vi "Queues Init.vi"(8 "error in (no error)":errorcluster, 11 "Guardian in":refnum<class "Guardian.lvclass">) -> (0 "error out":errorcluster, 3 "Guardian out":refnum<class "Guardian.lvclass">)   [LabVIEW 2026, in "TALOS.lvlib" / "Guardian.lvlib" / "Guardian.lvclass"]
uses:
  Guardian.lvclass
  Helper Loop Msg.ctl
  Helper Loop Msg Selector.ctl
  Guardian.lvclass/Guardian.ctl
  Ancestor/Ancestor/Ancestor.lvclass/Ancestor.ctl
  Support VIs/Generate Error.vi
  FGV/Error Memory/Get Error Description.vi
  Support VIs/Get PC name.vi
  Ancestor/Ancestor/Read ID.vi
  Support VIs/Get Class Name.vi
  <vilib>/Utility/error.llb/Clear Errors.vi
  FGV/Error Memory/Error Memory Core.vi
  <vilib>/AdvancedString/Delimited String to 1D String Array.vi
  <vilib>/AdvancedString/Delimited String to 1D String Array (string).vi
  Support VIs/Circus Root Path.vi
  FGV/Error Memory/Error Crt Lvl checker.vi
  FGV/Error Memory/Error Memory Core.vi/40c8088d-b597-4017-91af-faa98e00292e.vi
  FGV/Error Memory/Error Memory Core.vi/d4a3ab98-063c-4e44-b43d-fbdcfe6c2be2.vi
  Support VIs/Global Memory.vi
  <vilib>/Utility/LVClass/Get LV Class Name.vi
  Support VIs/Is in Packed Library.vi
  Support VIs/TALOS Root path.vi
  Support VIs/Read CSV worksheet.vi
  Support VIs/Global Constants.vi
  <vilib>/Utility/error.llb/General Error Handler.vi
  Support VIs/Error Log.vi
  Ancestor/Ancestor/Ancestor.lvclass
  <vilib>/Comparison/Equal/Equal Functor/Equal Functor.lvclass
  TALOS.lvlib
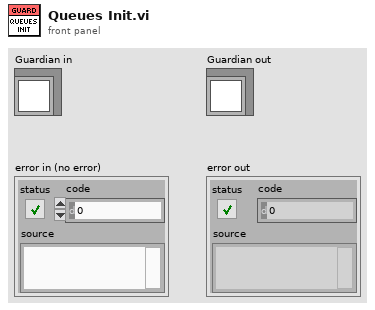
[diagram p1: front panel]
types:
  T1 = typedef "TALOS.lvlib/Guardian.lvlib/Guardian.lvclass/Helper Loop Msg.ctl" = cluster{"Helper Loop Msg Selector":T2, "Data":variant}
  T2 = typedef "TALOS.lvlib/Guardian.lvlib/Guardian.lvclass/Helper Loop Msg Selector.ctl" = enum16{"Test String"}
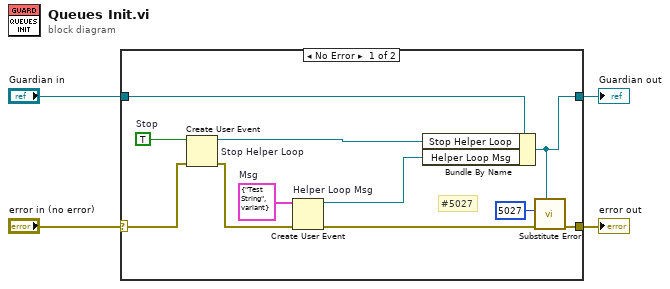
[diagram p0: block diagram]
diagram:
  n1 = case shown="No Error" "error in (no error)" {
    selector: "error in (no error)" -> [w13 w16]
    tunnel: [w6 w17] -> w4
    tunnel: [w7 w16] -> w3
    tunnel: "Guardian in" -> [w12 w17]
    frame No Error {
      w11 = T1 {"Helper Loop Msg Selector"=enum."Test String", "Data"=variant}  # Msg
      w14 = TRUE  # Stop
      # "#5027"
      n2 = Create User Event "Stop Helper Loop"(user event datatype=w14, error in=w13) -> (user event=w15:refnum<user-event>, error out=w10:errorcluster)
      n3 = Create User Event "Helper Loop Msg"(user event datatype=w11, error in=w10) -> (user event=w8:refnum<user-event>, error out=w9:errorcluster)
      n4 = Bundle By Name(cluster=w12, "Stop Helper Loop"=w15, "Helper Loop Msg"=w8) -> (w6:refnum<class "Guardian.lvclass">)
      n5 = call "Substitute Error.vi"("LabVIEW Object"=w6, "error in (no error)"=w9, "Error Code"=5027) -> ("error out"=w7:errorcluster)  [unwired: 8 in]
    }
    frame Error {
    }
  }
  "error out" <- w3
  "Guardian out" <- w4
